vi "Request Multiple DTCs.vi"(6 "Command":string, 8 "error in":errorcluster, 9 "Address":string, 10 "Lookup Table":variant, 11 "connection info":T4) -> (0 "error out":errorcluster, 1 "Responses":T3[](array[typedef]), 2 "Lookup Table Out":variant, 3 "connection info":T4, 4 "Error Array":T1[](array[typedef]))   [LabVIEW 2023, in "J1939 Addon Shared.lvlib"]
uses:
  J1939 Addon Shared.lvlib
  <vilib>/NI/STM/TCP/TCP Connection Info.ctl
  <vilib>/NI/STM/SubVIs/MetaDataElement.ctl
  Types/Convert DTCs Cluster.ctl
  Types/Error Cluster.ctl
  Types/Error Types.ctl
  Types/Address Lookup Table Data.ctl
  Types/Request Message.ctl
  <vilib>/NI/STM/NI STM.lvlib
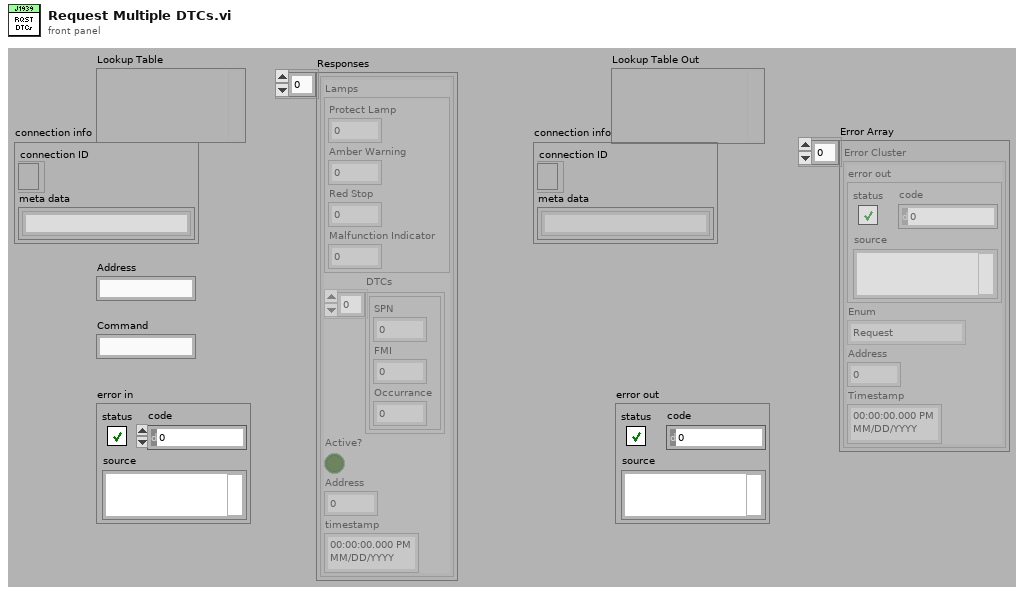
[diagram p1: front panel]
types:
  T1 = typedef "J1939 Addon Shared.lvlib/Error Cluster.ctl" = cluster{"error out":errorcluster, "Enum":T2, "Address":u8, "Timestamp":timestamp}
  T2 = typedef "J1939 Addon Shared.lvlib/Error Types.ctl" = enum16{"Request", "RAW Generation", "Clear Active DTCs", "Clear Previous DTCs", "Addresses", "TLAs", "Get Active DTCs", "Get Previous DTCs", "TCP Connection"}
  T3 = typedef "J1939 Addon Shared.lvlib/Convert DTCs Cluster.ctl" = cluster{"Lamps":cluster{"Protect Lamp":u8, "Amber Warning":u8, "Red Stop":u8, "Malfunction Indicator":u8}, "DTCs":cluster{"SPN":u32, "FMI":u8, "Occurrance":u8}[], "Active?":bool, "Address":u8, "timestamp":timestamp}
  T4 = typedef "NI STM.lvlib/TCP Connection Info.ctl" = cluster{"connection ID":refnum<k5>, "meta data":T5[]}
  T5 = typedef "NI STM.lvlib/MetaDataElement.ctl" = string
  T6 = typedef "J1939 Addon Shared.lvlib/Address Lookup Table Data.ctl" = cluster{"Name":u8[], "Address":u8}
  T7 = typedef "J1939 Addon Shared.lvlib/Request Message.ctl" = cluster{"PGN":u32, "DA":u8, "Ignore Response":bool}
  T8 = typedef "XNET Frame CAN.ctl" = cluster{"timestamp":timestamp, "payload":u8[], "identifier":u32, "type":T9, "extended?":bool, "echo?":bool}
  T9 = typedef "XNET Frame Type CAN.ctl" = u8
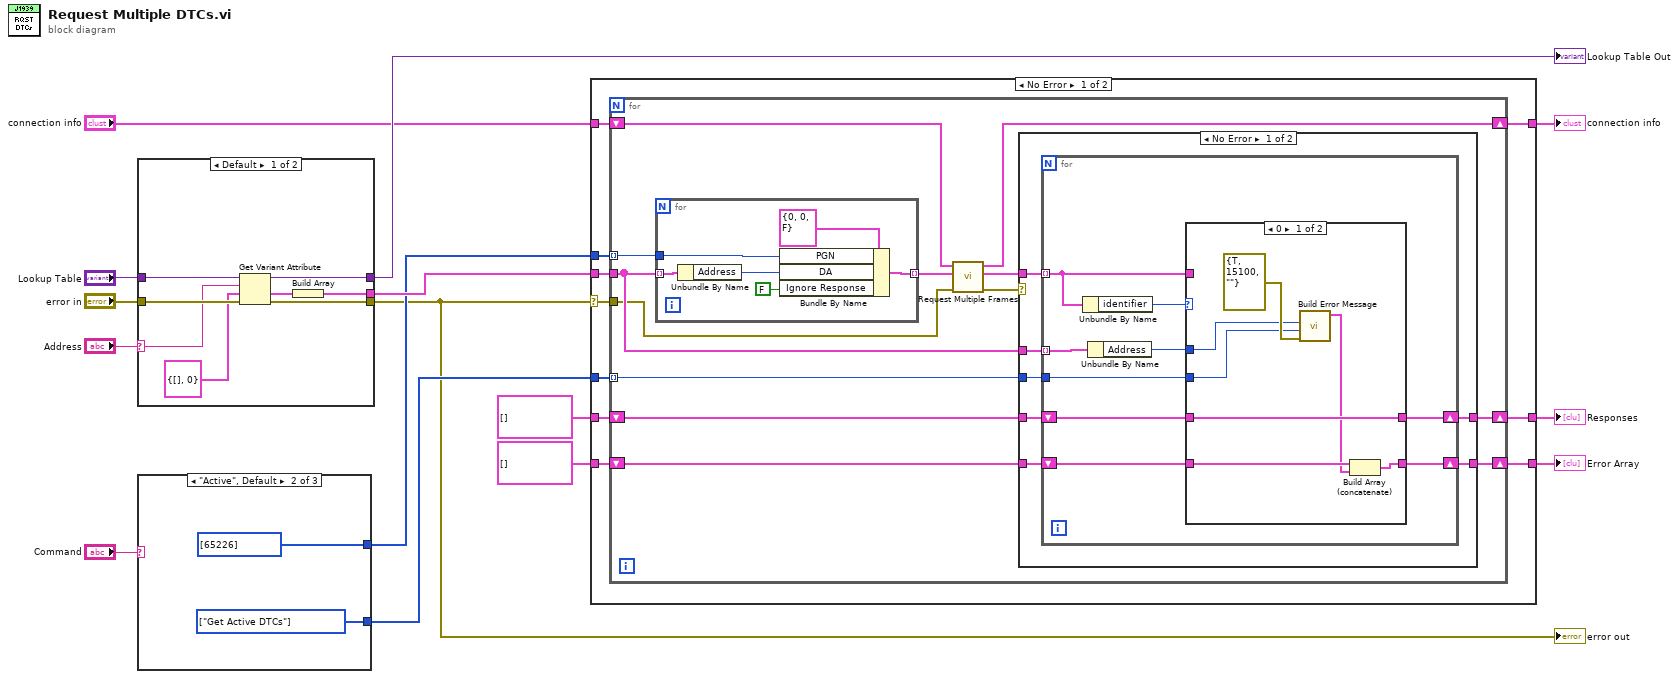
[diagram p0: block diagram]
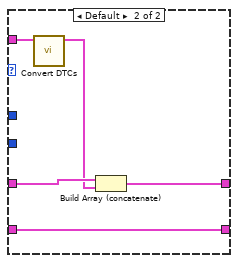
[diagram p2: hidden frame]
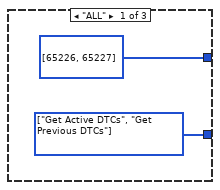
[diagram p5: hidden frame]
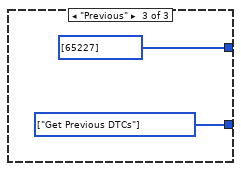
[diagram p6: hidden frame]
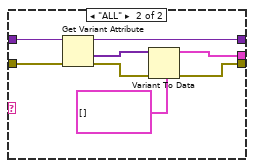
[diagram p7: hidden frame]
diagram:
  n1 = case shown="Default" "Address" {
    selector: "Address" -> [w18 _]
    tunnel: [w17 w24] -> w9
    tunnel: [w22 w31] -> w12
    tunnel: "Lookup Table" -> [w21 w30]
    tunnel: "error in" -> [w20 w29]
    tunnel: [w19 w27] -> w1
    frame Default {
      n2 = Get Variant Attribute(Variant=w21, name=w18, default value (empty Variant)=T6 {"Name"=[], "Address"=0} ("Data"), error in=w20) -> (duplicate Variant=w22:variant, value=w23:T6, error out=w19:errorcluster)  [unwired: 1 out]
      n3 = Build Array(w23) -> (w17:T6[])
    }
    frame "ALL" {
      n4 = Get Variant Attribute(Variant=w30, error in=w29) -> (duplicate Variant=w31:variant, values=w25:variant[], error out=w28:errorcluster)  [unwired: 2 in, 1 out]
      n5 = Variant To Data(error in=w28, type=T6[] [], Variant=w25) -> (data=w24:T6[], error out=w27:errorcluster)
    }
  }
  "Lookup Table Out" <- w12
  "error out" <- w1
  n6 = case shown="\"Active\", Default" "Command" {
    tunnel: [u32[] [65226, 65227] u32[] [65226] u32[] [65227]] -> w8
    tunnel: [w32 w34 w36] -> w7
    frame "ALL" {
      w32 = T2[] [enum."Get Active DTCs", enum."Get Previous DTCs"] items=["Request", "RAW Generation", "Clear Active DTCs", "Clear Previous DTCs", "Addresses", "TLAs", "Get Active DTCs", "Get Previous DTCs", "TCP Connection"]
    }
    frame "Active", Default {
      w34 = T2[] [enum."Get Active DTCs"] items=["Request", "RAW Generation", "Clear Active DTCs", "Clear Previous DTCs", "Addresses", "TLAs", "Get Active DTCs", "Get Previous DTCs", "TCP Connection"]
    }
    frame "Previous" {
      w36 = T2[] [enum."Get Previous DTCs"] items=["Request", "RAW Generation", "Clear Active DTCs", "Clear Previous DTCs", "Addresses", "TLAs", "Get Active DTCs", "Get Previous DTCs", "TCP Connection"]
    }
  }
  n7 = case shown="No Error" w1 {
    selector: w1 -> [w38 _]
    tunnel: "connection info" -> [w47 w97]
    tunnel: w9 -> [w46 _]
    tunnel: w8 -> [w45 _]
    tunnel: w7 -> [w44 _]
    tunnel: T3[] [] -> [w43 w98]
    tunnel: T1[] [] -> [w42 w99]
    tunnel: [w41 w97] -> w4
    tunnel: [w40 w98] -> w3
    tunnel: [w39 w99] -> w2
    frame No Error {
      n8 = for {
        tunnel: w46 -> [w56]
        tunnel: w45 -> [w55] mode=indexing
        tunnel: w44 -> [w54] mode=indexing
        shift-right: [w52] -> w40
        shift-left: w43 -> [w53]
        shift-right: [w50] -> w39
        shift-left: w42 -> [w51]
        shift-right: [w49] -> w41
        shift-left: w47 -> [w59]
        tunnel: w38 -> [w48]
        n9 = for {
          tunnel: w56 -> [w95] mode=indexing
          tunnel: [w92] -> w60 mode=indexing
          tunnel: w55 -> [w91]
          n10 = Unbundle By Name(w95) -> ("Address"=w94:u8)
          n11 = Bundle By Name(cluster=T7 {"PGN"=0, "DA"=0, "Ignore Response"=FALSE} ("Cluster"), "PGN"=w91, "DA"=w94, "Ignore Response"=FALSE) -> (w92:T7)
        }
        n12 = call "Request Multiple Frames.vi"("error in (no error)"=w48, "Requests"=w60, "connection info"=w59) -> ("error out"=w58:errorcluster, "Response Frames"=w57:T8[], "connection info"=w49:T4)  [unwired: 6 in]
        n13 = case shown="No Error" w58 {
          tunnel: w57 -> [w67 _]
          tunnel: w53 -> [w66 w89]
          tunnel: w51 -> [w65 w90]
          tunnel: w56 -> [w64 _]
          tunnel: w54 -> [w63 _]
          tunnel: [w62 w89] -> w52
          tunnel: [w61 w90] -> w50
          frame No Error {
            n14 = for {
              tunnel: w67 -> [w75] mode=indexing
              shift-right: [w73] -> w62
              shift-left: w66 -> [w74]
              shift-right: [w71] -> w61
              shift-left: w65 -> [w72]
              tunnel: w64 -> [w70] mode=indexing
              tunnel: w63 -> [w68]
              n15 = Unbundle By Name(w75) -> ("identifier"=w76:u32)
              n16 = Unbundle By Name(w70) -> ("Address"=w69:u8)
              n17 = case shown="0" w76 {
                tunnel: w75 -> [_ w88]
                tunnel: w74 -> [w83 w87]
                tunnel: [w83 w85] -> w73
                tunnel: w68 -> [w81 _]
                tunnel: w69 -> [w80 _]
                tunnel: w72 -> [w79 w84]
                tunnel: [w77 w84] -> w71
                frame 0 {
                  n18 = call "Build Error Message.vi"("error IO"=errorcluster {"status"=TRUE, "code"=15100, "source"=""}, "Enum"=w81, "Address"=w80) -> ("Error Cluster"=w78:T1)  [unwired: 8 in]
                  n19 = Build Array (concatenate)(w79, w78) -> (w77:T1[])
                }
                frame Default {
                  n20 = call "Convert DTCs.vi"("value"=w88) -> ("Cluster"=w86:T3)  [unwired: 10 in]
                  n21 = Build Array (concatenate)(w87, w86) -> (w85:T3[])
                }
              }
            }
          }
          frame Error {
          }
        }
      }
    }
    frame Error {
    }
  }
  "connection info" <- w4
  "Responses" <- w3
  "Error Array" <- w2
